vi "HP 34401 Read.vi"(2 "Point #":i32, 3 "Instrument Address":refnum<visa-resource-name>) -> (0 "Stop":bool, 1 "Measurement":dbl[](array[numeric]) format="%.6e")   [LabVIEW 2020]
doc: "This VI reads a single reading from a Keithley 2001 multimeter. The stop boolean is always false. If no reading is obtained a single zero is returned.\nScott Hannahs, NHMFL-FSU, Nov 1993"
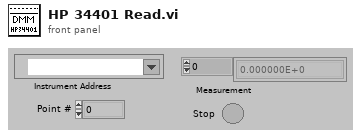
[diagram p1: front panel]
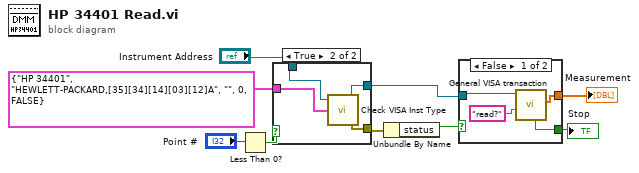
[diagram p0: block diagram]
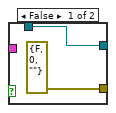
[diagram p2: hidden frame]
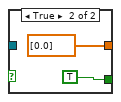
[diagram p3: hidden frame]
diagram:
  n1 = Less Than 0?(x="Point #") -> (x < 0?=w7:bool)
  n2 = case shown="True" w7 {
    tunnel: [w11 w15] -> w4
    tunnel: "Instrument Address" -> [w11 w13]
    tunnel: [errorcluster {"status"=FALSE, "code"=0, "source"=""} ("error out") w12] -> w1
    tunnel: cluster{string, string, string, u32, bool} {"HP 34401", "HEWLETT-PACKARD,[35][34][14][03][12]A", "", 0, FALSE} -> [_ w14]
    frame False {
    }
    frame True {
      n3 = call "Check VISA Inst Type.vi"("Check Parameters"=w14, "VISA session"=w13) -> ("Error Out"=w12:errorcluster, "dup VISA session"=w15:refnum<visa-resource-name>)  [unwired: 1 in, 1 out]
    }
  }
  n4 = Unbundle By Name(w1) -> ("status"=w2:bool)
  n5 = case shown="False" w2 {
    tunnel: w4 -> [w18 _]
    tunnel: [w17 dbl[] [0.0]] -> w8
    tunnel: [w16 TRUE ("Stop")] -> w9
    frame False {
      n6 = call "General VISA transaction.vi"("Command String"="read?", "VISA Session"=w18) -> ("Measurement"=w17:dbl[], "Stop"=w16:bool)  [unwired: 4 in, 4 out]
    }
    frame True {
    }
  }
  "Stop" <- w9
  "Measurement" <- w8
